vi "Write Temperature Controller.vi"(8 "error in (no error)":errorcluster, 10 "Temperature Controller":refnum<vi>, 11 "Function UI in":refnum<class "Controller UI.lvclass">) -> (0 "error out":errorcluster, 3 "Function UI out":refnum<class "Controller UI.lvclass">)   [LabVIEW 2016, in "Controller UI.lvlib" / "Controller UI.lvclass"]
uses:
  <userlib>/Common Components/Controller UI/Controller UI.lvclass
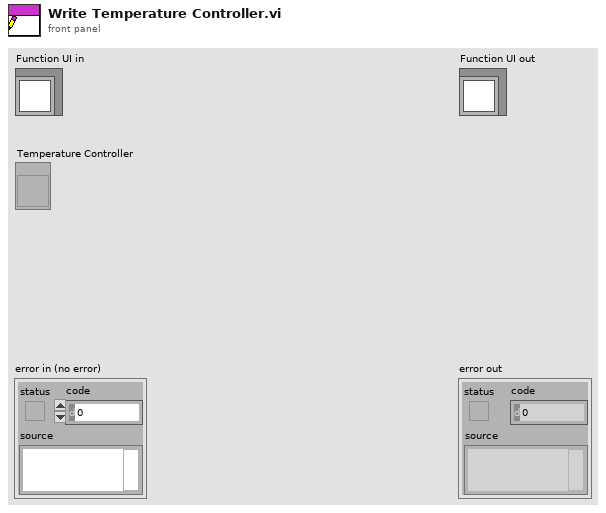
[diagram p1: front panel]
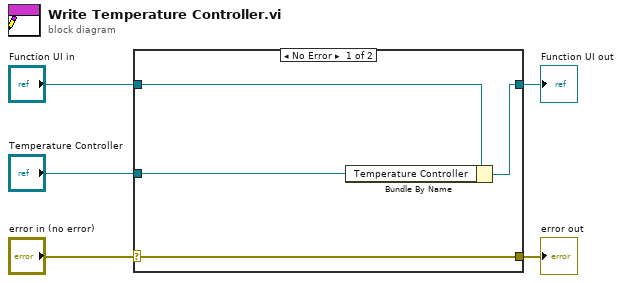
[diagram p0: block diagram]
diagram:
  n1 = case shown="No Error" "error in (no error)" {
    selector: "error in (no error)" -> [w9 w10]
    tunnel: [w9 w10] -> w4
    tunnel: [w7 w11] -> w2
    tunnel: "Function UI in" -> [w8 w11]
    tunnel: "Temperature Controller" -> [w6 _]
    frame No Error {
      n2 = Bundle By Name(cluster=w8, "Temperature Controller"=w6) -> (w7:refnum<class "Controller UI.lvclass">)
    }
    frame Error {
    }
  }
  "error out" <- w4
  "Function UI out" <- w2
